vi "TestEnsureIgorStringFormat.vi"(8 "error in (no error)":errorcluster) -> (0 "error out":errorcluster)   [LabVIEW 2016]
uses:
  <vilib>/addons/_JKI Toolkits/Caraya/classes/Test/Test.lvclass
  <vilib>/addons/_JKI Toolkits/Caraya/classes/Assert/Assert.lvclass
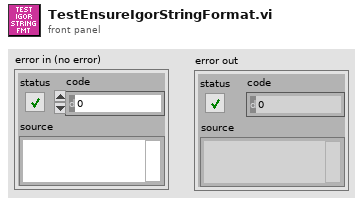
[diagram p1: front panel]
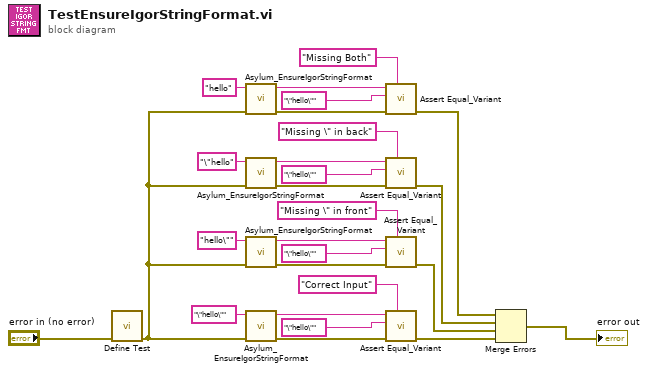
[diagram p0: block diagram]
diagram:
  n1 = call <vilib>:"Define Test.vi"("error in (no error)"="error in (no error)") -> ("error out"=w3:errorcluster)  [unwired: 10 in]
  n2 = call "Asylum_EnsureIgorStringFormat.vi"("error in (no error)"=w3, "Value"="hello") -> ("error out"=w13:errorcluster, "Value"=w12:string)  [unwired: 8 in]
  n3 = call "Asylum_EnsureIgorStringFormat.vi"("error in (no error)"=w3, "Value"="\"hello") -> ("error out"=w4:errorcluster, "Value"=w5:string)  [unwired: 8 in]
  n4 = call "Asylum_EnsureIgorStringFormat.vi"("error in (no error)"=w3, "Value"="hello\"") -> ("error out"=w15:errorcluster, "Value"=w16:string)  [unwired: 8 in]
  n5 = call "Asylum_EnsureIgorStringFormat.vi"("error in (no error)"=w3, "Value"="\"hello\"") -> ("error out"=w25:errorcluster, "Value"=w23:string)  [unwired: 8 in]
  n6 = call <vilib>:"Assert Equal_Variant.vi"("Label"="Missing Both", "error in (no error)"=w13, "Y"="\"hello\"" ("Value"), "X"=w12) -> ("error out"=w1:errorcluster)  [unwired: 7 in]
  n7 = call <vilib>:"Assert Equal_Variant.vi"("Label"="Missing \" in back", "error in (no error)"=w4, "Y"="\"hello\"" ("Value"), "X"=w5) -> ("error out"=w2:errorcluster)  [unwired: 7 in]
  n8 = call <vilib>:"Assert Equal_Variant.vi"("Label"="Missing \" in front", "error in (no error)"=w15, "Y"="\"hello\"" ("Value"), "X"=w16) -> ("error out"=w14:errorcluster)  [unwired: 7 in]
  n9 = call <vilib>:"Assert Equal_Variant.vi"("Label"="Correct Input", "error in (no error)"=w25, "Y"="\"hello\"" ("Value"), "X"=w23) -> ("error out"=w24:errorcluster)  [unwired: 7 in]
  n10 = Merge Errors(w1, w2, w14, w24) -> (→"error out":errorcluster)
